vi "Grab  with Callbacks.vi"(11 "uSerialNumber IN":u32=953000216) -> ()   [LabVIEW 2014]
uses:
  <vilib>/addons/PixeLINK/Low Level Functions/TRANSLATION.llb/TDPU-Translation-CallbacksInfo.ctl
  <vilib>/addons/PixeLINK/Low Level Functions/TRANSLATION.llb/TDPU-Translation-CallBackFlags.ctl
  <vilib>/addons/PixeLINK/Low Level Functions/ACQUISITION.llb/TDPU-Acquisition-StreamState.ctl
  <vilib>/addons/PixeLINK/Low Level Functions/CAMERA_FEATURES.llb/TDPU-CameraFeatures-FeatureIds.ctl
  <vilib>/addons/PixeLINK/Low Level Functions/CAMERA_FEATURES.llb/TDPU-CameraFeatures-FeatureFlags.ctl
panel:
  in  "stop":bool
  in  "CallbacksInfo":T1 {"uOverlayUse" items=["OVERLAY_PREVIEW             0x01", "OVERLAY_FORMAT_IMAGE  0x02", "OVERLAY_FORMAT_CLIP     0x04", "OVERLAY_FRAME                 0x08"]}
  # "This VI initializes the camera and starts the preview.  It also calls an overlay callback which draws a cross-hair on the preview window.\nIt works best with a color camera.\n\nBe sure to use the STOP button to allow the application to properly clean up and exit."
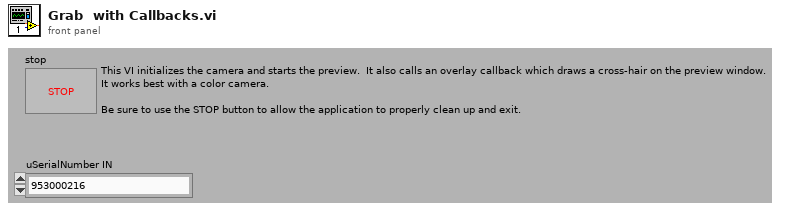
[diagram p1: front panel]
types:
  T1 = typedef "TDPU-Translation-CallbacksInfo.ctl" = cluster{"Occurrence":refnum<k4>, "hCamera":u32, "uOverlayUse":T2, "Path":path, "bGetClip":bool, "uNumberofFrameCaptured":u32, "error (Get Clip) ":errorcluster, "TerminationOccurence":refnum<k4>, "PDS Clip Path":path, "AVI Clip Path":path}
  T2 = typedef "TDPU-Translation-CallBackFlags.ctl" = u32
  T3 = typedef "TDPU-CameraFeatures-FeatureFlags.ctl" = u32
  T4 = typedef "TDPU-CameraFeatures-FeatureIds.ctl" = u32
  T5 = typedef "TDPU-Acquisition-StreamState.ctl" = u32
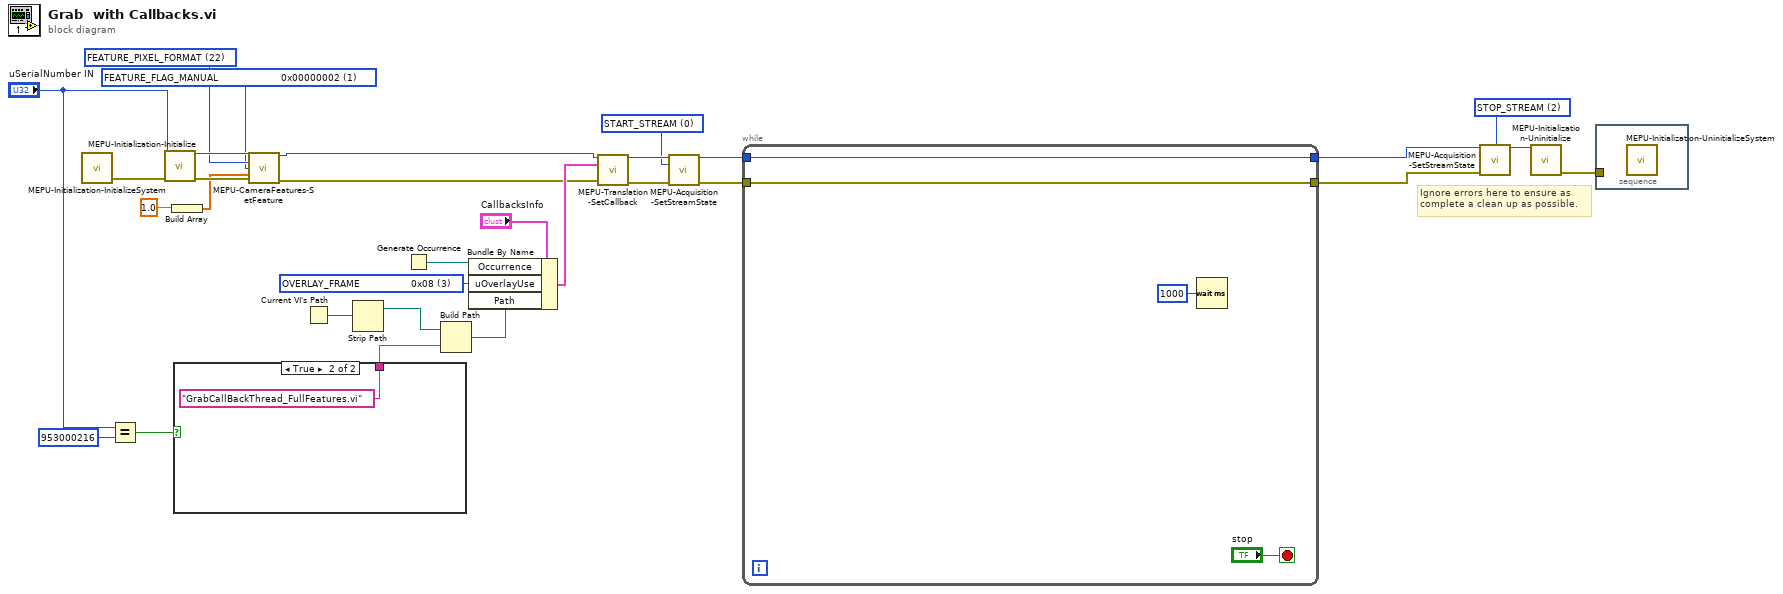
[diagram p0: block diagram]
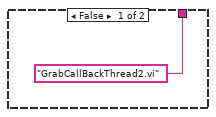
[diagram p2: hidden frame]
diagram:
  w7 = T3 1 items=["FEATURE_FLAG_PRESENCE                 0x00000001", "FEATURE_FLAG_MANUAL                     0x00000002", "FEATURE_FLAG_AUTO                         0x00000004", "FEATURE_FLAG_ONEPUSH                   0x00000008", "FEATURE_FLAG_OFF                            0x00000010", "FEATURE_FLAG_DESC_SUPPORTED    0x00000020", "FEATURE_FLAG_READ_ONLY               0x00000040"] ("uFlags IN")
  w8 = T4 22 items=["FEATURE_BRIGHTNESS", "FEATURE_EXPOSURE", "FEATURE_SHARPNESS", "FEATURE_WHITE_BAL", "FEATURE_HUE", "FEATURE_SATURATION", "FEATURE_GAMMA", "FEATURE_SHUTTER", "FEATURE_GAIN", "FEATURE_IRIS", "FEATURE_FOCUS", "FEATURE_TEMPERATURE", "FEATURE_TRIGGER", "FEATURE_ZOOM", "FEATURE_PAN", "FEATURE_TILT", "FEATURE_OPT_FILTER", "FEATURE_GPIO", "FEATURE_FRAME_RATE", "FEATURE_ROI", "FEATURE_FLIP", "FEATURE_PIXEL_ADDRESSING", "FEATURE_PIXEL_FORMAT", "FEATURE_EXTENDED_SHUTTER", "FEATURE_AUTO_ROI", "FEATURE_LOOKUP_TABLE", "FEATURE_MEMORY_CHANNEL", "FEATURE_WHITE_SHADING", "FEATURE_ROTATE", "FEATURE_IMAGER_CLK_DIVISOR", "FEATURE_TRIG_WITH_CNTRLD_LIGHT", "FEATURE_MAX_PIXEL_SIZE"] ("uFeatureId IN")
  w18 = T5 2 items=["START_STREAM", "PAUSE_STREAM", "STOP_STREAM"] ("uStreamState IN")
  w23 = T2 3 items=["OVERLAY_PREVIEW             0x01", "OVERLAY_FORMAT_IMAGE  0x02", "OVERLAY_FORMAT_CLIP     0x04", "OVERLAY_FRAME                 0x08"] ("uOverlayUse")
  w25 = T5 0 items=["START_STREAM", "PAUSE_STREAM", "STOP_STREAM"] ("uStreamState IN")
  # "Ignore errors here to ensure as\ncomplete a clean up as possible."
  n1 = call <vilib>:"MEPU-Initialization-InitializeSystem.vi"() -> ("Error OUT"=w30:errorcluster)  [unwired: 15 in]
  n2 = Equal?(x="uSerialNumber IN", y=u32 953000216) -> (x = y?=w13:bool)
  n3 = call <vilib>:"MEPU-Initialization-Initialize.vi"("uSerialNumber IN"="uSerialNumber IN", "Error IN"=w30) -> ("phCamera OUT"=w12:u32, "Error OUT"=w9:errorcluster)  [unwired: 11 in, 1 out]
  n4 = Build Array(1.0) -> (w5:dbl[])
  n5 = case shown="True" w13 {
    tunnel: ["GrabCallBackThread2.vi" ("name or relative path") "GrabCallBackThread_FullFeatures.vi" ("name or relative path")] -> w20
    frame False {
    }
    frame True {
    }
  }
  n6 = call <vilib>:"MEPU-CameraFeatures-SetFeature.vi"("hCamera IN"=w12, "uFeatureId IN"=w8, "uFlags IN"=w7, "pParms IN"=w5, "Error IN"=w9) -> ("hCamera OUT"=w11:u32, "Error OUT"=w10:errorcluster)  [unwired: 8 in, 1 out]
  n7 = Current VI's Path() -> (path=w22:path)
  n8 = Strip Path(path=w22) -> (stripped path=w21:path)  [unwired: 1 out]
  n9 = Generate Occurrence() -> (w24:refnum<k4>)
  n10 = Build Path(base path=w21, name or relative path=w20) -> (appended path=w19:path)
  n11 = Bundle By Name(cluster="CallbacksInfo", "Occurrence"=w24, "uOverlayUse"=w23, "Path"=w19) -> (w28:T1)
  n12 = call <vilib>:"MEPU-Translation-SetCallback.vi"("hCamera IN"=w11, "CallbackInfo IN"=w28, "Error IN"=w10) -> ("hCamera OUT"=w26:u32, "Error OUT"=w27:errorcluster)  [unwired: 10 in, 1 out]
  n13 = call <vilib>:"MEPU-Acquisition-SetStreamState.vi"("hCamera IN"=w26, "uStreamState IN"=w25, "Error IN"=w27) -> ("hCamera OUT"=w4:u32, "Error OUT"=w2:errorcluster)  [unwired: 11 in]
  n14 = while {
    tunnel: w4 -> [w34]
    tunnel: [w34] -> w3
    tunnel: w2 -> [w33]
    tunnel: [w33] -> w1
    stop <- "stop" stop-if-true
    n15 = Wait (ms)(milliseconds to wait=u32 1000) -> ()  [unwired: 1 out]
  }
  n16 = call <vilib>:"MEPU-Acquisition-SetStreamState.vi"("hCamera IN"=w3, "uStreamState IN"=w18, "Error IN"=w1) -> ("hCamera OUT"=w16:u32)  [unwired: 11 in, 1 out]
  n17 = call <vilib>:"MEPU-Initialization-Uninitialize.vi"("hCamera IN"=w16) -> ("Error OUT"=w17:errorcluster)  [unwired: 14 in]
  n18 = stacked-sequence {
    tunnel: w17 -> [_]
    frame #0 {
      n19 = call <vilib>:"MEPU-Initialization-UninitializeSystem.vi"() -> ()  [unwired: 15 in, 1 out]
    }
  }
